vi "ParseErrors.vi"(8 "ErrorArray":errorcluster[](array[cluster])) -> (0 "ErrorArray":errorcluster[](array[cluster]), 1 "Severity":string[](array[string]), 2 "Priority":i32[](array[numeric]))   [LabVIEW 2014, in "NISTErrorLib.lvlib"]
uses:
  NISTErrorLib.lvlib
panel:
  # "Sorts the Error Array and extracts Priority and Severity Info.\nOutputs a sorted error array, priority array, and severity array"
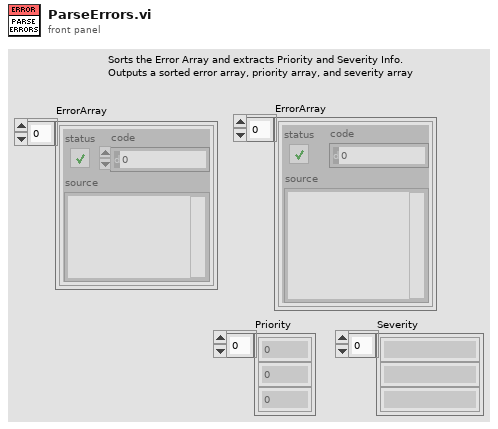
[diagram p1: front panel]
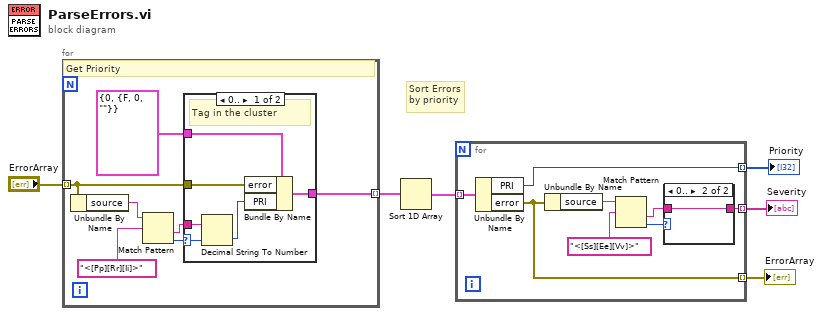
[diagram p0: block diagram]
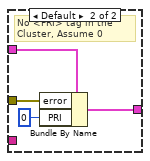
[diagram p3: hidden frame]
diagram:
  # "Sort Errors\nby priority"
  n1 = for {
    tunnel: "ErrorArray" -> [w11] mode=indexing
    tunnel: [w10] -> w5 mode=indexing
    # "Get Priority"
    n2 = Unbundle By Name(w11) -> ("source"=w12:string)
    n3 = Match Pattern(string=w12, regular expression="<[Pp][Rr][Ii]>") -> (after substring=w8:string, offset past match=w13:i32)  [unwired: 1 in, 2 out]
    n4 = case shown="0.." w13 {
      selector: w13 -> [w16 _]
      tunnel: w11 -> [w19 w23]
      tunnel: [w18 w21] -> w10
      tunnel: w8 -> [w15 _]
      tunnel: cluster{"PRI":i32, "error":errorcluster} {"PRI"=0, "error"={"status"=FALSE, "code"=0, "source"=""}} -> [w14 w20]
      frame 0.. {
        # "Tag in the cluster"
        n5 = Decimal String To Number(string=w15, default (0L)=w16) -> (number=w17:i32)  [unwired: 1 in, 1 out]
        n6 = Bundle By Name(cluster=w14, "error"=w19, "PRI"=w17) -> (w18:cluster{"PRI":i32, "error":errorcluster})
      }
      frame Default {
        # "No <PRI> tag in the Cluster, Assume 0"
        n7 = Bundle By Name(cluster=w20, "error"=w23, "PRI"=0) -> (w21:cluster{"PRI":i32, "error":errorcluster})
      }
    }
  }
  n8 = Sort 1D Array(array=w5) -> (sorted array=w4:cluster{"PRI":i32, "error":errorcluster}[])
  n9 = for {
    tunnel: w4 -> [w31] mode=indexing
    tunnel: [w30] -> w3 mode=indexing
    tunnel: [w29] -> w2 mode=indexing
    tunnel: [w25] -> w1 mode=indexing
    n10 = Unbundle By Name(w31) -> ("PRI"=w30:i32, "error"=w29:errorcluster)
    n11 = Unbundle By Name(w29) -> ("source"=w27:string)
    n12 = Match Pattern(string=w27, regular expression="<[Ss][Ee][Vv]>") -> (after substring=w24:string, offset past match=w26:i32)  [unwired: 1 in, 2 out]
    n13 = case shown="0.." w26 {
      tunnel: w24 -> [_ w32]
      tunnel: [_ w32] -> w25
      frame Default {
      }
      frame 0.. {
      }
    }
  }
  "Priority" <- w3
  "ErrorArray" <- w2
  "Severity" <- w1
